vi "AD7747_Setup.vi"(8 "error in":errorcluster, 10 "AD7747_Number":string="900D80", 11 "Control":refnum<visa-resource-name>) -> (0 "error out":errorcluster, 3 "Control out":refnum<visa-resource-name>, 4 "Data Out":string[](array[string]))   [LabVIEW 2017]
panel:
  # "AD7747 Setup for Cap Measurements"
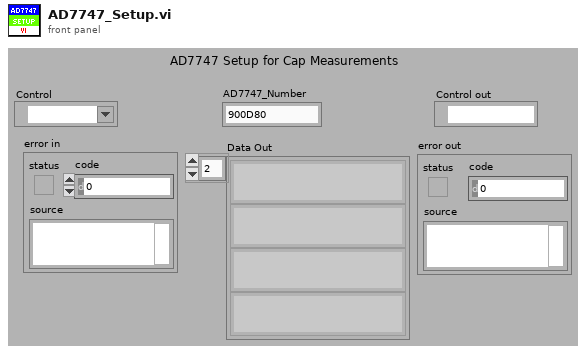
[diagram p1: front panel]
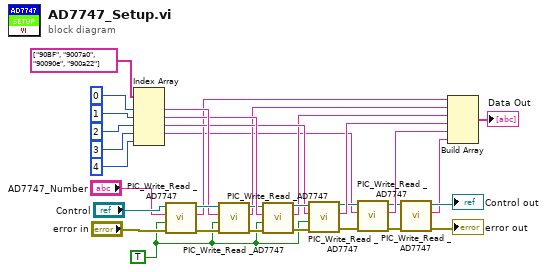
[diagram p0: block diagram]
diagram:
  w10 = TRUE ("Time Delay")
  n1 = Index Array(array=string[] ["90BF", "9007a0", "90090e", "900a22"], index #1=0 ("index"), index #2=1 ("index"), index #3=2 ("index"), index #4=3 ("index"), index #5=4 ("index")) -> (element #1=w26:string, element #2=w25:string, element #3=w21:string, element #4=w7:string)  [unwired: 1 out]
  n2 = call "PIC_Write_Read _AD7747.vi"("error in (no error)"="error in", "Time Delay"=w10, "command"="AD7747_Number", "Control"="Control") -> ("error out"=w29:errorcluster, "output"=w16:string, "Control out"=w28:refnum<visa-resource-name>)  [unwired: 5 in]
  n3 = call "PIC_Write_Read _AD7747.vi"("error in (no error)"=w29, "Time Delay"=w10, "command"=w26, "Control"=w28) -> ("error out"=w27:errorcluster, "output"=w15:string, "Control out"=w24:refnum<visa-resource-name>)  [unwired: 5 in]
  n4 = call "PIC_Write_Read _AD7747.vi"("error in (no error)"=w27, "Time Delay"=w10, "command"=w25, "Control"=w24) -> ("error out"=w23:errorcluster, "output"=w14:string, "Control out"=w22:refnum<visa-resource-name>)  [unwired: 5 in]
  n5 = call "PIC_Write_Read _AD7747.vi"("error in (no error)"=w23, "Time Delay"=w10, "command"=w21, "Control"=w22) -> ("error out"=w9:errorcluster, "output"=w13:string, "Control out"=w8:refnum<visa-resource-name>)  [unwired: 5 in]
  n6 = call "PIC_Write_Read _AD7747.vi"("error in (no error)"=w9, "command"=w7, "Control"=w8) -> ("error out"=w6:errorcluster, "output"=w5:string, "Control out"=w4:refnum<visa-resource-name>)  [unwired: 6 in]
  n7 = call "PIC_Write_Read _AD7747.vi"("error in (no error)"=w6, "Control"=w4) -> ("error out"=→"error out":errorcluster, "output"=w1:string, "Control out"=→"Control out":refnum<visa-resource-name>)  [unwired: 7 in]
  n8 = Build Array(w16, w15, w14, w13, w5, w1) -> (→"Data Out":string[])
